vi "Write Graphs refs.vi"(8 "error in (no error)":errorcluster, 10 "Graph refs":T1, 11 "Control-Client in":refnum<class "Control-Client.lvclass">) -> (0 "error out":errorcluster, 3 "Control-Client out":refnum<class "Control-Client.lvclass">)   [LabVIEW 2018, in "Control-Client.lvclass"]
uses:
  Control-Client.lvclass
  dependecies/ControlsVIs/Clusters-def/Graphs_ref_Client.ctl
  dependecies/ControlsVIs/Clusters-def/graphs_TR.ctl
  Control-Client.lvclass/Control-Client.ctl
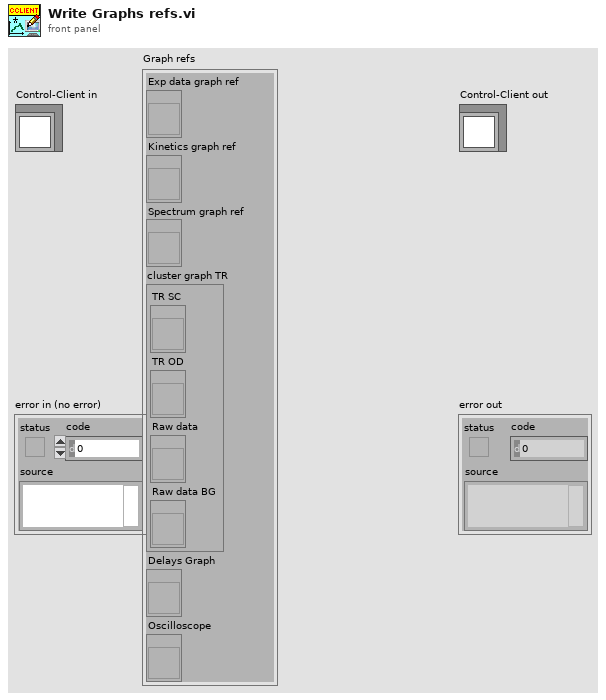
[diagram p1: front panel]
types:
  T1 = typedef "Control-Client.lvclass/Graphs_ref_Client.ctl" = cluster{"Exp data graph ref":refnum<vi>, "Kinetics graph ref":refnum<vi>, "Spectrum graph ref":refnum<vi>, "cluster graph TR":T2, "Delays Graph":refnum<vi>, "Oscilloscope":refnum<vi>}
  T2 = typedef "graphs_TR.ctl" = cluster{"TR SC":refnum<vi>, "TR OD":refnum<vi>, "Raw data":refnum<vi>, "Raw data BG":refnum<vi>}
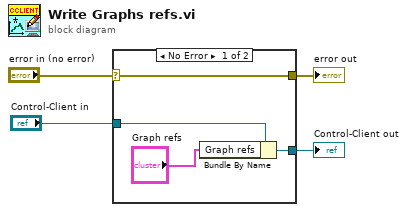
[diagram p0: block diagram]
diagram:
  n1 = case shown="No Error" "error in (no error)" {
    selector: "error in (no error)" -> [w8 w9]
    tunnel: [w8 w9] -> w3
    tunnel: [w6 w10] -> w1
    tunnel: "Control-Client in" -> [w7 w10]
    frame No Error {
      n2 = Bundle By Name(cluster=w7, "Graph refs"="Graph refs") -> (w6:refnum<class "Control-Client.lvclass">)
    }
    frame Error {
    }
  }
  "error out" <- w3
  "Control-Client out" <- w1
